vi "Decode_Modbus_Message.vi"(8 "error in (no error)":errorcluster, 9 "E_values":T2) -> (0 "error out":errorcluster, 1 "E_values 2":T2)   [LabVIEW 2026]
panel:
  in  "Mensaje":T1
  out "E_muneca":u32(knob) scale=0.0..400.0
  out "E_antebrazo":u32(knob) scale=0.0..400.0
  out "E_codo":u32(knob) scale=0.0..400.0
  out "E_hombro":u32(knob) scale=0.0..400.0
  out "E_cadera":u32(knob) scale=0.0..400.0
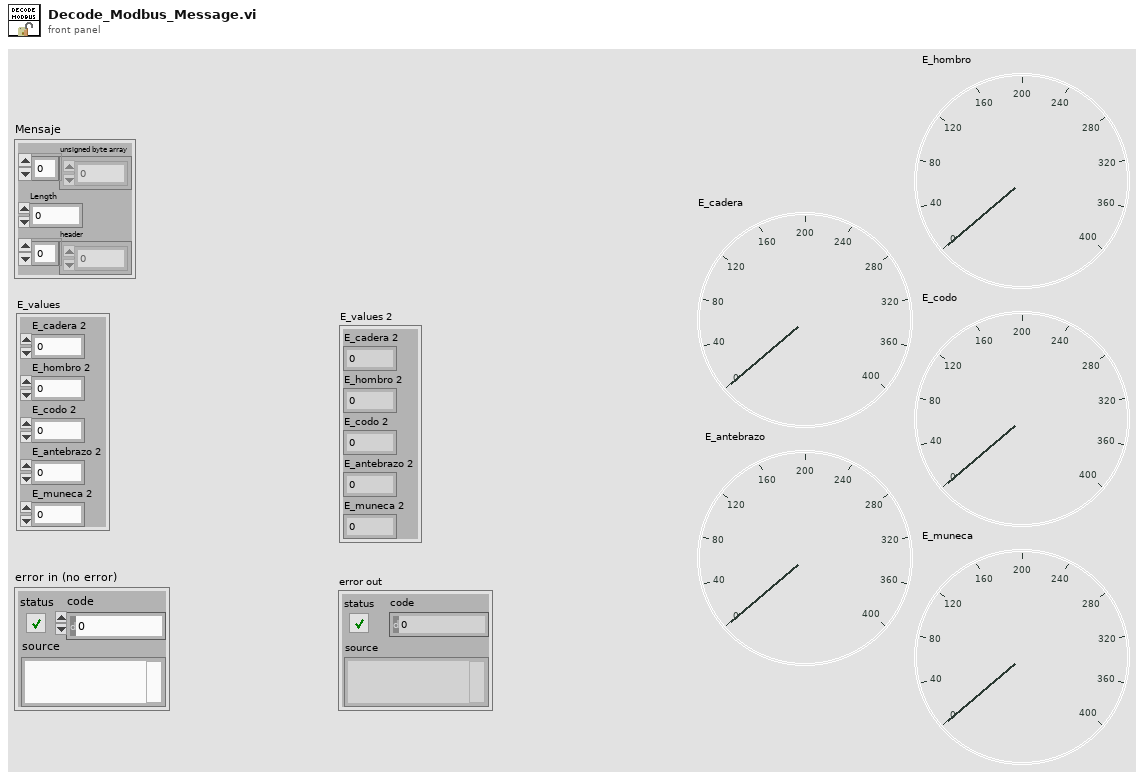
[diagram p1: front panel]
types:
  T1 = cluster{"unsigned byte array":u8[], "Length":u8, "header":u8[]}
  T2 = cluster{"E_cadera 2":u32, "E_hombro 2":u32, "E_codo 2":u32, "E_antebrazo 2":u32, "E_muneca 2":u32}
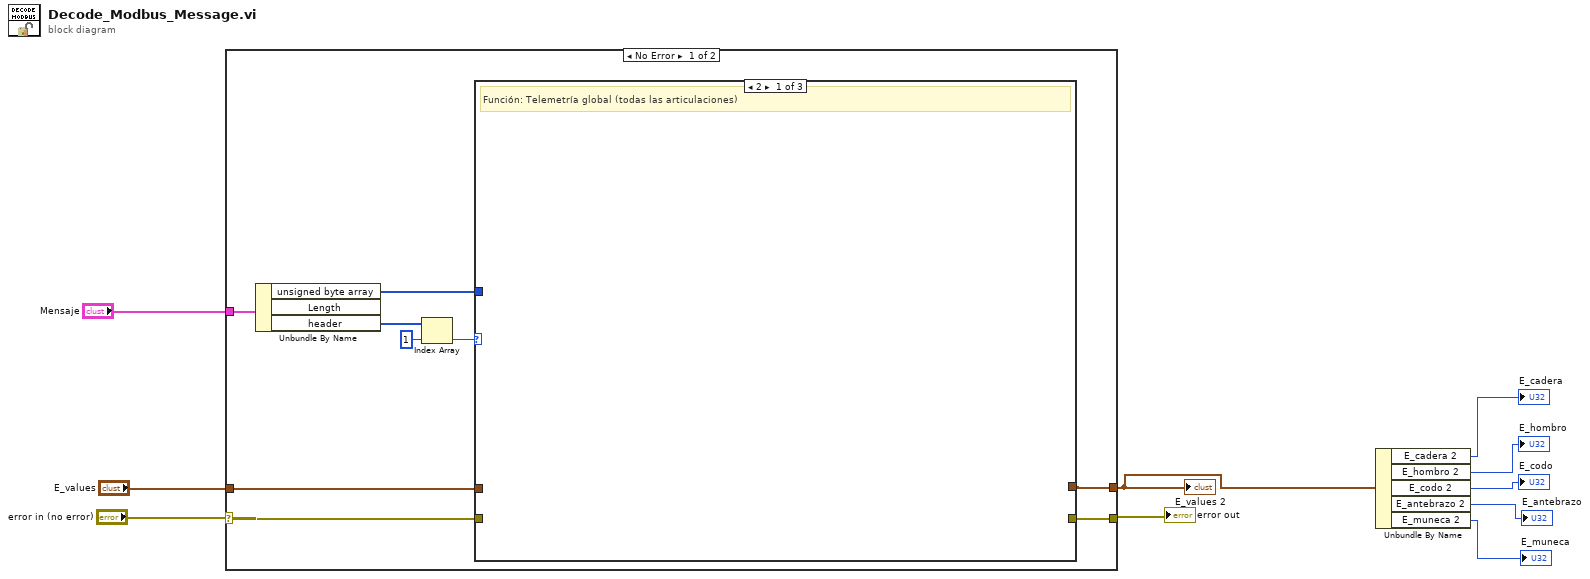
[diagram p0: block diagram]
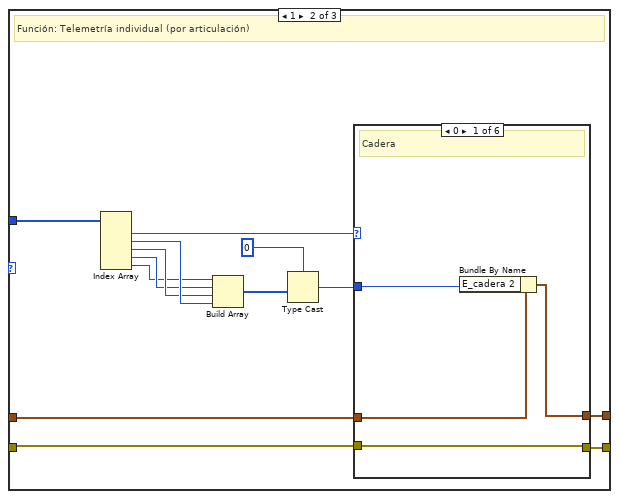
[diagram p2: hidden frame]
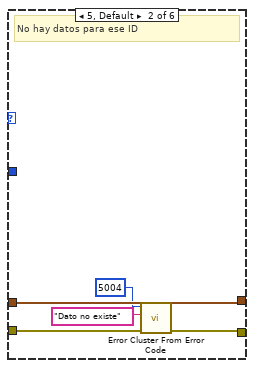
[diagram p3: hidden frame]
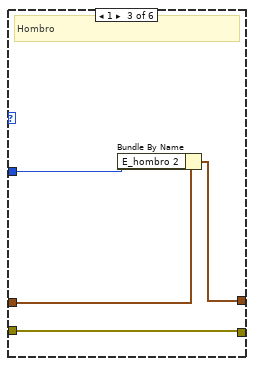
[diagram p4: hidden frame]
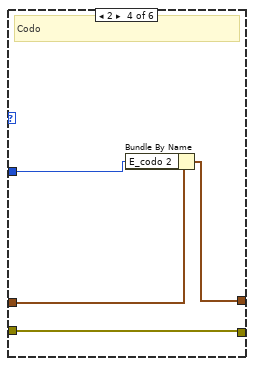
[diagram p5: hidden frame]
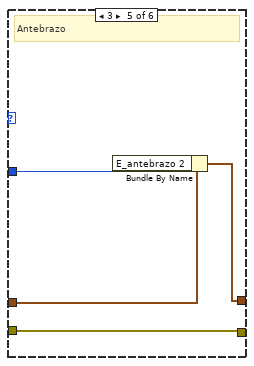
[diagram p6: hidden frame]
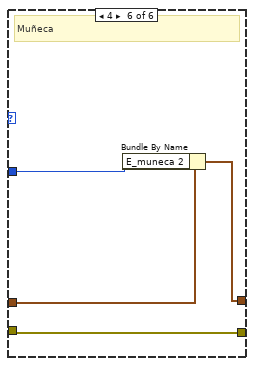
[diagram p7: hidden frame]
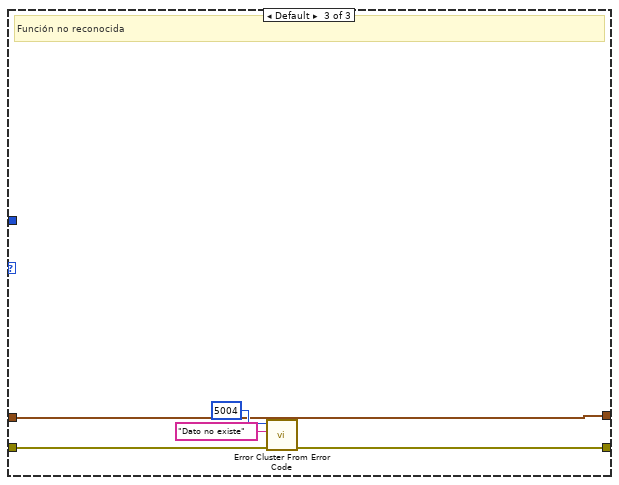
[diagram p8: hidden frame]
diagram:
  n1 = case shown="No Error" "error in (no error)" {
    selector: "error in (no error)" -> [w15 w63]
    tunnel: "E_values" -> [w13 w64]
    tunnel: "Mensaje" -> [w19 _]
    tunnel: [w14 w63] -> w7
    tunnel: [w12 w64] -> w6
    frame No Error {
      n2 = Unbundle By Name(w19) -> ("unsigned byte array"=w11:u8[], "header"=w17:u8[])  [unwired: 1 out]
      n3 = Index Array(array=w17, index=1) -> (element=w16:u8)
      n4 = case shown="2" w16 {
        tunnel: w15 -> [_ w20 w60]
        tunnel: [_ w21 w59] -> w14
        tunnel: w13 -> [_ w29 w58]
        tunnel: [_ w28 w58] -> w12
        tunnel: w11 -> [_ w27 _]
        frame 2 {
          # "Función: Telemetría global (todas las articulaciones)"
        }
        frame 1 {
          # "Función: Telemetría individual (por articulación)"
          n5 = Index Array(array=w27) -> (element #1=w26:u8, element #2=w25:u8, element #3=w24:u8, element #4=w23:u8, element #5=w22:u8)  [unwired: 5 in]
          n6 = Build Array(w22, w23, w24, w25) -> (w31:u8[])
          n7 = Type Cast(type=u32 0, x=w31) -> (*(type *) &x=w32:u32)
          n8 = case shown="0" w26 {
            tunnel: [w36 w41 w45 w48 w52 w56] -> w28
            tunnel: w32 -> [w35 _ w44 w49 w53 w57]
            tunnel: w29 -> [w34 w41 w43 w47 w51 w55]
            tunnel: [w33 w38 w42 w46 w50 w54] -> w21
            tunnel: w20 -> [w33 w37 w42 w46 w50 w54]
            frame 0 {
              # "Cadera"
              n9 = Bundle By Name(cluster=w34, "E_cadera 2"=w35) -> (w36:T2)
            }
            frame 5, Default {
              # "No hay datos para ese ID"
              n10 = call <vilib>:"Error Cluster From Error Code.vi"("error in (no error)"=w37, "error message (\"\")"="Dato no existe" ("error message (\"\")"), "error code (0)"=5004) -> ("error out"=w38:errorcluster)  [unwired: 6 in]
            }
            frame 1 {
              # "Hombro"
              n11 = Bundle By Name(cluster=w43, "E_hombro 2"=w44) -> (w45:T2)
            }
            frame 2 {
              # "Codo"
              n12 = Bundle By Name(cluster=w47, "E_codo 2"=w49) -> (w48:T2)
            }
            frame 3 {
              # "Antebrazo"
              n13 = Bundle By Name(cluster=w51, "E_antebrazo 2"=w53) -> (w52:T2)
            }
            frame 4 {
              # "Muñeca"
              n14 = Bundle By Name(cluster=w55, "E_muneca 2"=w57) -> (w56:T2)
            }
          }
        }
        frame Default {
          # "Función no reconocida"
          n15 = call <vilib>:"Error Cluster From Error Code.vi"("error in (no error)"=w60, "error message (\"\")"="Dato no existe" ("error message (\"\")"), "error code (0)"=5004) -> ("error out"=w59:errorcluster)  [unwired: 6 in]
        }
      }
    }
    frame Error {
    }
  }
  "error out" <- w7
  "E_values 2" <- w6
  n16 = Unbundle By Name(w6) -> ("E_cadera 2"=→"E_cadera":u32, "E_hombro 2"=→"E_hombro":u32, "E_codo 2"=→"E_codo":u32, "E_antebrazo 2"=→"E_antebrazo":u32, "E_muneca 2"=→"E_muneca":u32)
